vi "ShooterPID.vi"(10 "Current":dbl, 11 "Set":dbl) -> (3 "Shooter Motor":dbl)   [LabVIEW 2012]
uses:
  <vilib>/addons/control/pid/pid.llb/PID (DBL).vi
  <vilib>/addons/control/pid/NI_PID_pid.lvlib
panel:
  in  "PID gains":T1={"proportional gain (Kc)"=1.0, "integral time (Ti, min)"=0.01, "derivative time (Td, min)"=0.0} {"derivative time (Td, min)" format="%.3f"; "integral time (Ti, min)" format="%.3f"; "proportional gain (Kc)" format="%.3f"}
  out "Error":dbl(graph)
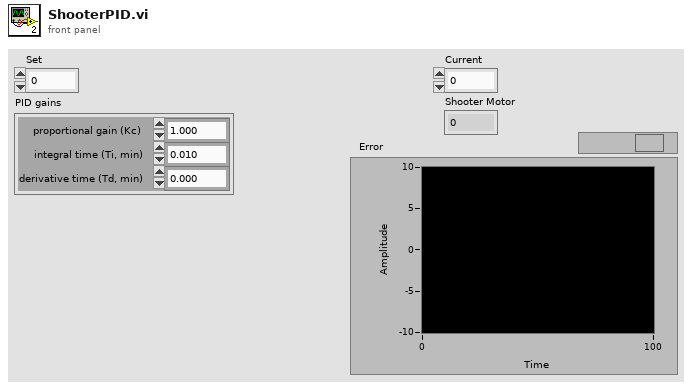
[diagram p1: front panel]
types:
  T1 = cluster{"proportional gain (Kc)":dbl, "integral time (Ti, min)":dbl, "derivative time (Td, min)":dbl}
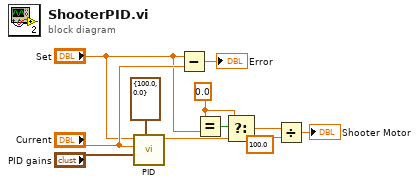
[diagram p0: block diagram]
diagram:
  w4 = 0.0 ("y")
  n1 = call-poly <vilib>:"PID.vi"("output range"=cluster{"output high":dbl, "output low":dbl} {"output high"=100.0, "output low"=0.0}, "PID gains"="PID gains", "process variable"="Current", "setpoint"="Set") -> ("output"=w7:dbl)  [unwired: 6 in, 1 out]
  n2 = Subtract(x="Set", y="Current") -> (x-y=→"Error":dbl)
  n3 = Equal?(x=w4, y="Set") -> (x = y?=w3:bool)
  n4 = Select(t=w4, s=w3, f=w7) -> (s? t:f=w5:dbl)
  n5 = Divide(x=w5, y=100.0) -> (x/y=→"Shooter Motor":dbl)
